vi "Update Comparison Values.vi"(5 "Type":T1, 6 "Path":path, 7 "Operation":string, 8 "error in (no error)":errorcluster, 10 "Digits of Precision":u8) -> (0 "error out":errorcluster)   [LabVIEW 2016]
doc: "Changes the comparison values (High and Low Comparison values or just Comparison Value depending on the requested operation) digits of precision for floating point data types"
uses:
  <vilib>/Utility/Data Type/Type Definitions/Data Type.ctl
  <vilib>/Utility/Data Type/NI_Data Type.lvlib
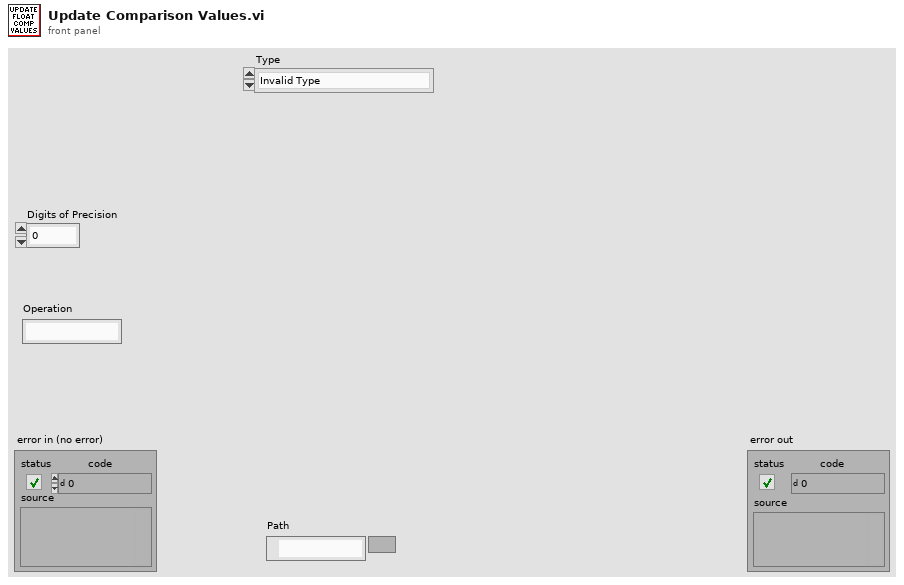
[diagram p1: front panel]
types:
  T1 = typedef "NI_Data Type.lvlib/Data Type.ctl" = enum8{"Invalid Type", "Void", "I8", "I16", "I32", "I64", "U8", "U16", "U32", "U64", "Single Float", "Double Float", "Extended Float", "Single Complex", "Double Complex", "Extended Complex", "Enum U8", "Enum U16", "Enum U32", "Enum U64", "Single Float With Unit", "Double Float With Unit", "Extended Float With Unit", "Single Complex with Unit", "Double Complex with Unit", "Extended Complex with Unit", "Boolean", "String", "Path", "Picture", "Tag", "Array", "Cluster", "Variant", "LV Variant", "Waveform", "Timestamp", "Digital Waveform", "Digital Data", "ExpressData", "Refnum", "External Data", "VI", "Poly VI", "LabVIEW Class Instance", "Fixed Point"}
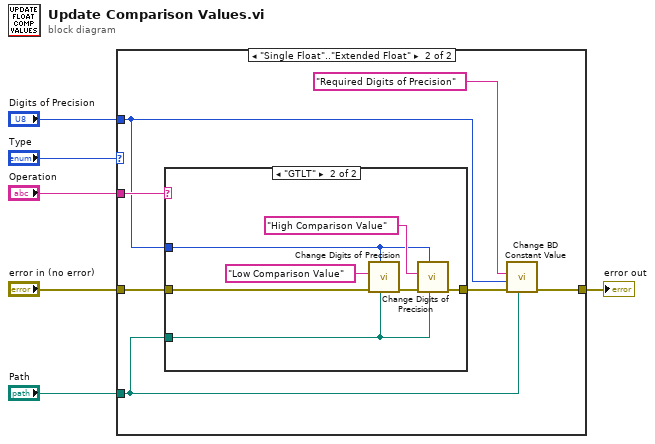
[diagram p0: block diagram]
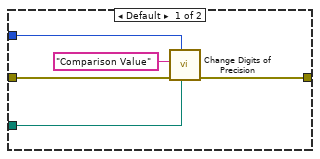
[diagram p3: hidden frame]
diagram:
  n1 = case shown="\"Single Float\"..\"Extended Float\"" "Type" {
    tunnel: "Operation" -> [_ w14]
    tunnel: "Path" -> [_ w10]
    tunnel: "Digits of Precision" -> [_ w8]
    tunnel: "error in (no error)" -> [w7 w13]
    tunnel: [w7 w11] -> w1
    frame Default {
      # "Do nothing to the digits of precision unless it is a floating point data type"
    }
    frame "Single Float".."Extended Float" {
      n2 = case shown="\"GTLT\"" w14 {
        tunnel: w10 -> [w16 w21]
        tunnel: w8 -> [w18 w24]
        tunnel: w13 -> [w17 w23]
        tunnel: [w15 w22] -> w12
        frame Default {
          n3 = call "Change Digits of Precision.vi"("VI Path"=w16, "Digits of Precision"=w18, "error in (no error)"=w17, "Numeric Constant Name"="Comparison Value" ("Constant Name")) -> ("error out"=w15:errorcluster)  [unwired: 7 in]
        }
        frame "GTLT" {
          n4 = call "Change Digits of Precision.vi"("VI Path"=w21, "Digits of Precision"=w24, "error in (no error)"=w23, "Numeric Constant Name"="Low Comparison Value" ("Constant Name")) -> ("error out"=w20:errorcluster)  [unwired: 7 in]
          n5 = call "Change Digits of Precision.vi"("VI Path"=w21, "Digits of Precision"=w24, "error in (no error)"=w20, "Numeric Constant Name"="High Comparison Value" ("Constant Name")) -> ("error out"=w22:errorcluster)  [unwired: 7 in]
        }
      }
      n6 = call "Change BD Constant Value.vi"("Assert VI Path"=w10, "error in (no error)"=w12, "Data Value"=w8, "Constant Name"="Required Digits of Precision") -> ("error out"=w11:errorcluster)  [unwired: 7 in]
    }
  }
  "error out" <- w1
